vi "I2C_MASTER_WRITE_NEW.vi"(1 "error in (no error)":errorcluster, 2 "Latch":bool, 3 "y Stepper value":u8, 4 "Arduino mode":T1) -> (0 "error out":errorcluster)   [LabVIEW 2018]
uses:
  I2C_MASTER_WRITE_NEW Type Def.ctl
  <vilib>/Studica/Studica Toolkit/Background/I2C Channel.ctl
panel:
  out "Data To Write":u8[](array[numeric])
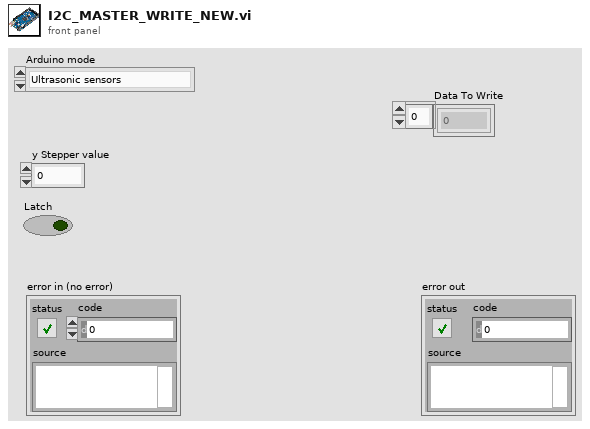
[diagram p1: front panel]
types:
  T1 = typedef "I2C_MASTER_WRITE_NEW Type Def.ctl" = enum16{"Ultrasonic sensors", "Stepper origin", "zStepper 13.3k", "zStepper 13k", "zStepper 12k", "zStepper 11k", "zStepper 10k", "zStepper 9k", "zStepper 8k", "zStepper 7k", "zStepper 6k", "zStepper 5k", "zStepper 4k", "zStepper 3k", "zStepper 2k", "zStepper 1k", "zStepper 900", "zStepper 800", "zStepper 700", "zStepper 600", "zStepper 500", "zStepper 400", "zStepper 300", "zStepper 200", "zStepper 100", "zStepper 0", "yStepper control", "Open Claw", "Close Claw", "Soft Reset"}
  T2 = typedef "I2C Channel.ctl" = enum16{"Not Connected", "A", "B"}
  T3 = cluster{"I2C Channel":T2, "FPGA VI Reference Out":refnum<k20>}
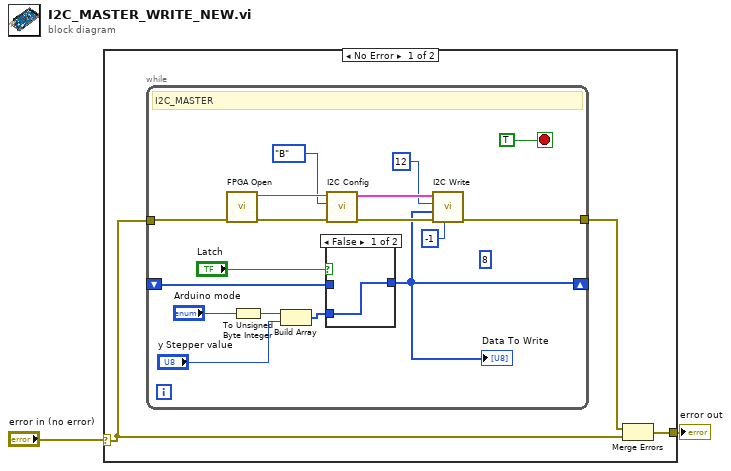
[diagram p0: block diagram]
diagram:
  n1 = case shown="No Error" "error in (no error)" {
    selector: "error in (no error)" -> [w4 w25]
    tunnel: [w5 w25] -> w1
    frame No Error {
      n2 = while {
        tunnel: w4 -> [w14]
        shift-right: [w11] -> _
        shift-left: _ -> [w9]
        tunnel: [w8] -> w3
        stop <- TRUE ("stop") stop-if-true
        (unwired) u32 8 ("Bytes to Read")
        # "I2C_MASTER"
        n3 = call <vilib>:"FPGA Open.vi"("error in (no error)"=w14) -> ("error out"=w20:errorcluster, "FPGA Reference Out"=w21:refnum<k20>)  [unwired: 9 in]
        n4 = To Unsigned Byte Integer(number="Arduino mode") -> (unsigned 8bit integer=w13:u8)
        n5 = Build Array(w13, "y Stepper value") -> (w12:u8[])
        n6 = case shown="False" "Latch" {
          tunnel: w12 -> [w23 _]
          tunnel: [w23 w24] -> w11
          tunnel: w9 -> [_ w24]
          frame False {
          }
          frame True {
          }
        }
        "Data To Write" <- w11
        n7 = call <vilib>:"I2C Config.vi"("error in (no error)"=w20, "I2C Channel"=I2C_Channel."B", "FPGA Reference"=w21) -> ("error out"=w17:errorcluster, "I2C Ref Out"=w18:T3)  [unwired: 7 in]
        n8 = call <vilib>:"I2C Write.vi"("Timeout ms (1000)"=-1, "error in (no error)"=w17, "Data to Write"=w11, "Slave Address (7-bit)"=u8 12, "I2C Ref In"=w18) -> ("error out"=w8:errorcluster)  [unwired: 5 in, 1 out]
      }
      n9 = Merge Errors(w3, w4) -> (w5:errorcluster)
    }
    frame Error {
    }
  }
  "error out" <- w1
